vi "PhotonMultiTargetPNPResult_Equals.vi"(9 "Other PhotonMultiTargetPNPResult":T1={"PhotonPNPResult"={"IsPresent"=FALSE, "bestReprojErr"=0.0, "altReprojErr"=0.0, "ambiguity"=0.0, "Best"={"TRANSLATION3D"={"X"=0.0, "Y"=0.0, "Z"=0.0}, "ROTATION3D"={"Q_quaternion"={"R"=1.0, "V"=[0.0, 0.0, 0.0]}}, "XF"=FALSE}, "Alt"={"TRANSLATION3D"={"X"=0.0, "Y"=0.0, "Z"=0.0}, "ROTATION3D"={"Q_quaternion"={"R"=1.0, "V"=[0.0, 0.0, 0.0]}}, "XF"=FALSE}}, "FiducialIDsUsed"=[]} {"PhotonPNPResult"."Alt"."TRANSLATION3D"."Z" format="%14.3f"; "PhotonPNPResult"."Alt"."TRANSLATION3D"."Y" format="%14.3f"; "PhotonPNPResult"."Alt"."TRANSLATION3D"."X" format="%14.3f"; "PhotonPNPResult"."Best"."TRANSLATION3D"."Z" format="%14.3f"; "PhotonPNPResult"."Best"."TRANSLATION3D"."Y" format="%14.3f"; "PhotonPNPResult"."Best"."TRANSLATION3D"."X" format="%14.3f"}, 11 "PhotonMultiTargetPNPResult":T1={"PhotonPNPResult"={"IsPresent"=FALSE, "bestReprojErr"=0.0, "altReprojErr"=0.0, "ambiguity"=0.0, "Best"={"TRANSLATION3D"={"X"=0.0, "Y"=0.0, "Z"=0.0}, "ROTATION3D"={"Q_quaternion"={"R"=1.0, "V"=[0.0, 0.0, 0.0]}}, "XF"=FALSE}, "Alt"={"TRANSLATION3D"={"X"=0.0, "Y"=0.0, "Z"=0.0}, "ROTATION3D"={"Q_quaternion"={"R"=1.0, "V"=[0.0, 0.0, 0.0]}}, "XF"=FALSE}}, "FiducialIDsUsed"=[]} {"PhotonPNPResult"."Alt"."TRANSLATION3D"."Z" format="%14.3f"; "PhotonPNPResult"."Alt"."TRANSLATION3D"."Y" format="%14.3f"; "PhotonPNPResult"."Alt"."TRANSLATION3D"."X" format="%14.3f"; "PhotonPNPResult"."Best"."TRANSLATION3D"."Z" format="%14.3f"; "PhotonPNPResult"."Best"."TRANSLATION3D"."Y" format="%14.3f"; "PhotonPNPResult"."Best"."TRANSLATION3D"."X" format="%14.3f"}) -> (3 "Equal":bool)   [LabVIEW 2019, in "PhotonVisionLib.lvlib"]
doc: "Determines if two PhotonMultiTargetPNPResult clusters are equal.\n\nInputs:\n - PhotonMultiTargetPNPResult -- PhotonMultiTargetPNPResult cluster.\n - OtherPhotonMultiTargetPNPResult -- OtherPhotonMultiTargetPNPResult cluster.\n\nOutputs:\n - Equal -- Returns TRUE, if both PhotonMultiTargetPNPResult clusters are equal.."
uses:
  PhotonVisionLib.lvlib
  <vilib>/Rock Robotics/WPI/ThirdParty/JAS_Junk/TrajLib/TypeDef/TRANSLATION3D.ctl
  <vilib>/Rock Robotics/WPI/ThirdParty/JAS_Junk/TrajLib/Trajectory_Library.lvlib
  <vilib>/Rock Robotics/WPI/ThirdParty/JAS_Junk/TrajLib/TypeDef/QUATERNION.ctl
  <vilib>/Rock Robotics/WPI/ThirdParty/JAS_Junk/TrajLib/TypeDef/ROTATION3D.ctl
  <vilib>/Rock Robotics/WPI/ThirdParty/JAS_Junk/TrajLib/TypeDef/TRANSFORM3D.ctl
  TypeDef/PhotonPNPResultType.ctl
  TypeDef/PhotonMultiTargetPNPResultType.ctl
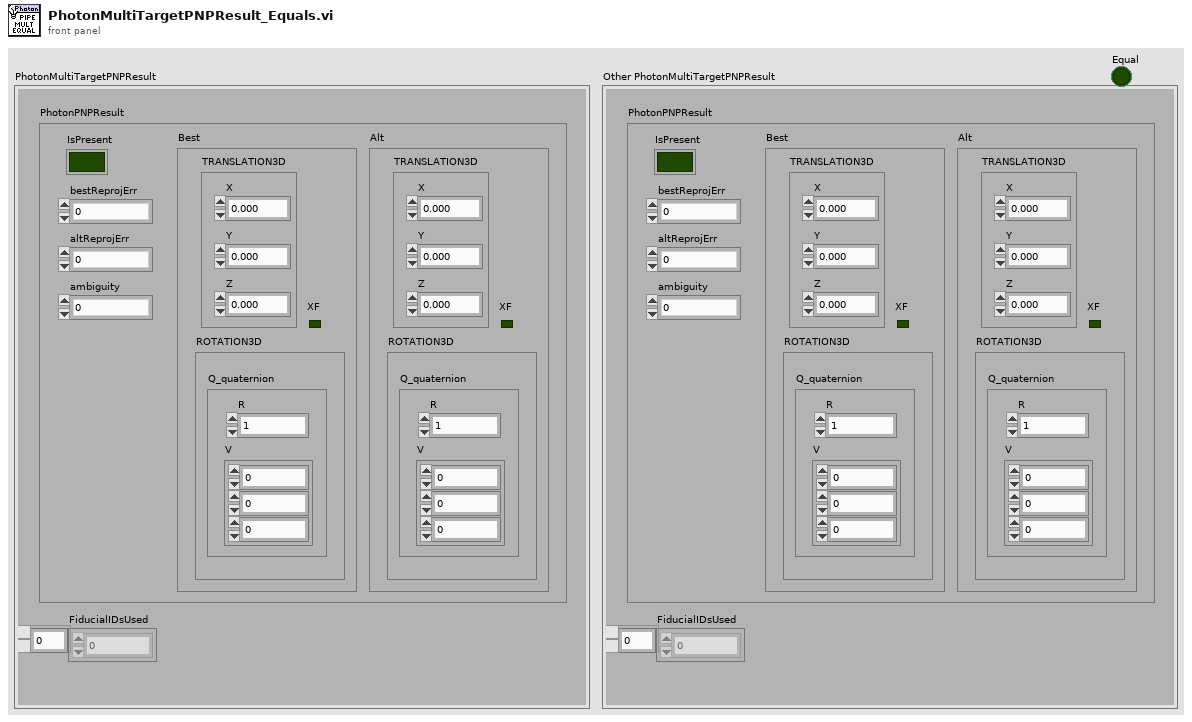
[diagram p1: front panel]
types:
  T1 = typedef "PhotonVisionLib.lvlib/PhotonMultiTargetPNPResultType.ctl" = cluster{"PhotonPNPResult":T2, "FiducialIDsUsed":i16[]}
  T2 = typedef "PhotonVisionLib.lvlib/PhotonPNPResultType.ctl" = cluster{"IsPresent":bool, "bestReprojErr":dbl, "altReprojErr":dbl, "ambiguity":dbl, "Best":T3, "Alt":T3}
  T3 = typedef "Trajectory_Library.lvlib/TRANSFORM3D.ctl" = cluster{"TRANSLATION3D":T4, "ROTATION3D":T5, "XF":bool}
  T4 = typedef "Trajectory_Library.lvlib/TRANSLATION3D.ctl" = cluster{"X":dbl, "Y":dbl, "Z":dbl}
  T5 = typedef "Trajectory_Library.lvlib/ROTATION3D.ctl" = cluster{"Q_quaternion":T6}
  T6 = typedef "Trajectory_Library.lvlib/QUATERNION.ctl" = cluster{"R":dbl, "V":dbl[]}
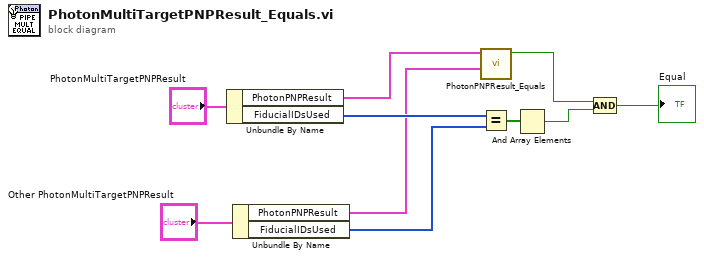
[diagram p0: block diagram]
diagram:
  n1 = Unbundle By Name("PhotonMultiTargetPNPResult") -> ("PhotonPNPResult"=w3:T2, "FiducialIDsUsed"=w8:i16[])
  n2 = Unbundle By Name("Other PhotonMultiTargetPNPResult") -> ("PhotonPNPResult"=w2:T2, "FiducialIDsUsed"=w7:i16[])
  n3 = call "PhotonPNPResult_Equals.vi"("Other PhotonPNPResult"=w2, "PhotonPNPResult"=w3) -> ("Equal"=w1:bool)  [unwired: 9 in]
  n4 = Equal?(x=w8, y=w7) -> (x = y?=w6:bool[])
  n5 = And Array Elements(Boolean array=w6) -> (logical AND=w5:bool)
  n6 = Compound Arithmetic op=AND(w1, w5) -> (→"Equal":bool)
